vi "imu.vi"(4 "error in":errorcluster) -> (0 "error out":errorcluster, 1 "IMU configuration":string, 2 "Raw data":string, 3 "IMU Packet":T1 {"local_angular_velocity"."z" format="%#.4g"; "local_angular_velocity"."y" format="%#.4g"; "local_angular_velocity"."x" format="%#.4g"; "angular_acceleration"."z" format="%#.3g"; "angular_acceleration"."y" format="%#.3g"; "angular_acceleration"."x" format="%#.3g"; "orientation"."w" format="%#.4g"; "orientation"."z" format="%#.4g"; "orientation"."y" format="%#.4g"; "orientation"."x" format="%#.4g"; "position"."z" format="%#_5g"; "position"."y" format="%#_5g"; "position"."x" format="%#_5g"; "local_velocity"."z" format="%#.4g"; "local_velocity"."y" format="%#.4g"; "local_velocity"."x" format="%#.4g"; "local_acceleration"."z" format="%#.4g"; "local_acceleration"."y" format="%#.4g"; "local_acceleration"."x" format="%#.4g"; "velocity"."z" format="%#.3g"; "velocity"."y" format="%#.3g"; "velocity"."x" format="%#.3g"; "angular_velocity"."z" format="%#.4g"; "angular_velocity"."y" format="%#.4g"; "angular_velocity"."x" format="%#.4g"; "acceleration"."z" format="%#.4g"; "acceleration"."y" format="%#.4g"; "acceleration"."x" format="%#.4g"})   [LabVIEW 2019]
doc: "Reads and process the data stream for the IMU sensor. Outputs the IMU data in a cluster."
uses:
  tools/simx_common.vi
  controls/IMU_packet.ctl
  controls/Header.ctl
panel:
  out "Header":T2 {"game_time" format="%#_10g"}
  in  "IMU configuration":string="{\n    \"type\": \"IMU\",\n    \"listen_port\": 8500,\n    \"location\": {\n      \"x\": 50.0,\n      \"y\": 50.0,\n      \"z\": 50.0\n    },\n    \"rotation\": {\n      \"pitch\":0.0,\n      \"yaw\":0.0,\n      \"roll\":0.0\n    }\n  }"
  in  "null connection":refnum<k5>
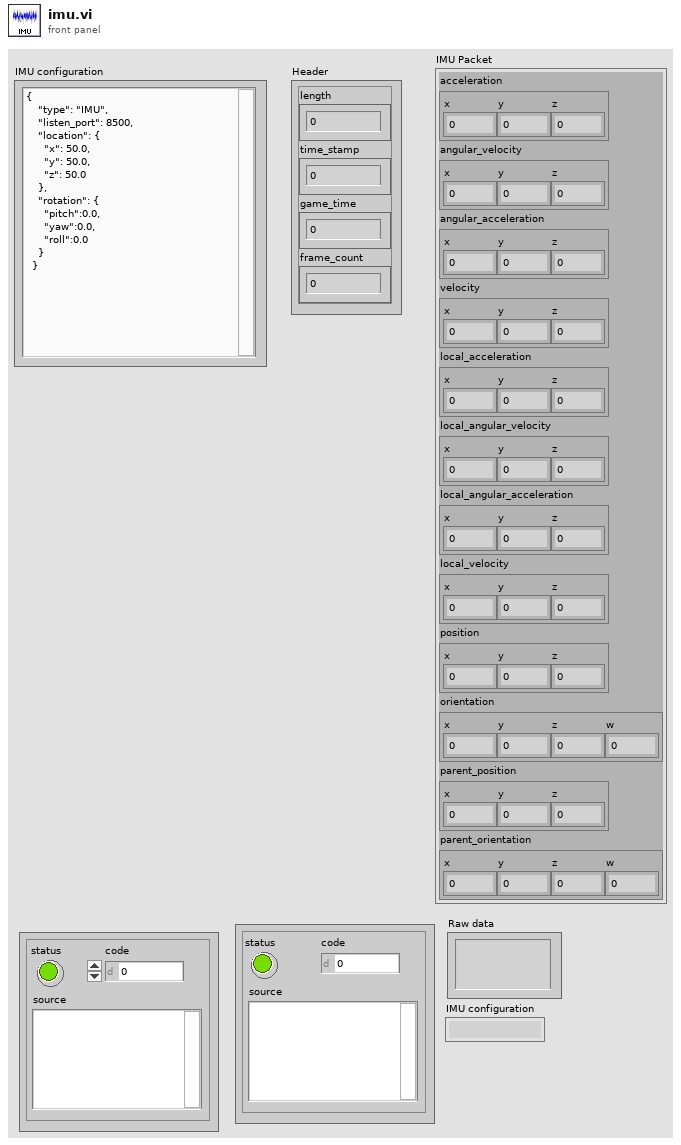
[diagram p1: front panel]
types:
  T1 = typedef "IMU_packet.ctl" = cluster{"acceleration":cluster{"x":sgl, "y":sgl, "z":sgl}, "angular_velocity":cluster{"x":sgl, "y":sgl, "z":sgl}, "angular_acceleration":cluster{"x":sgl, "y":sgl, "z":sgl}, "velocity ":cluster{"x":sgl, "y":sgl, "z":sgl}, "local_acceleration":cluster{"x":sgl, "y":sgl, "z":sgl}, "local_angular_velocity":cluster{"x":sgl, "y":sgl, "z":sgl}, "local_angular_acceleration":cluster{"x":sgl, "y":sgl, "z":sgl}, "local_velocity":cluster{"x":sgl, "y":sgl, "z":sgl}, "position":cluster{"x":sgl, "y":sgl, "z":sgl}, "orientation":cluster{"x":sgl, "y":sgl, "z":sgl, "w":sgl}, "parent_position":cluster{"x":sgl, "y":sgl, "z":sgl}, "parent_orientation":cluster{"x":sgl, "y":sgl, "z":sgl, "w":sgl}}
  T2 = typedef "Header.ctl" = cluster{"length":u32, "time_stamp":u32, "game_time":sgl, "frame_count":u32}
  T3 = typedef "simx_connection.ctl" = cluster{"Config":T4, "Connections":T7, "Map":cluster{"lanes":cluster{"x":dbl[], "y":dbl[], "z":dbl[]}, "StartPosition":cluster{"start_points":T8, "StartRotation":dbl[], "StartLocation":dbl[]}, "Draw Map Size":T9, "DrawArea":cluster{"min_Y":dbl, "min_X":dbl, "Scale X":dbl, "Scale Y":dbl}, "Map":picture, "Map Geojson":string}}
  T4 = typedef "config.ctl" = cluster{"Trajectory":T5, "Weather":T6}
  T5 = typedef "trajectory.ctl" = cluster{"Number of frames":i32, "Frame number":i32, "Trajectory":string}
  T6 = typedef "weather.ctl" = cluster{"id":string}
  T7 = typedef "connections.ctl" = cluster{"Simulator Connection":refnum<k5>, "server_ip":string, "Port":i32, "Sensor connections":refnum<k5>[]}
  T8 = typedef "start_points.ctl" = cluster{"locations":dbl[][], "rotations":dbl[][], "type":string[]}
  T9 = typedef "LVBoundsTypeDef.ctl" = cluster{"Width":u32, "Height":u32}
  T10 = enum16{"big-endian, network order", "native, host order", "little-endian"}
  T11 = typedef "sensor_sample.ctl" = cluster{"Header":T2, "data out":string}
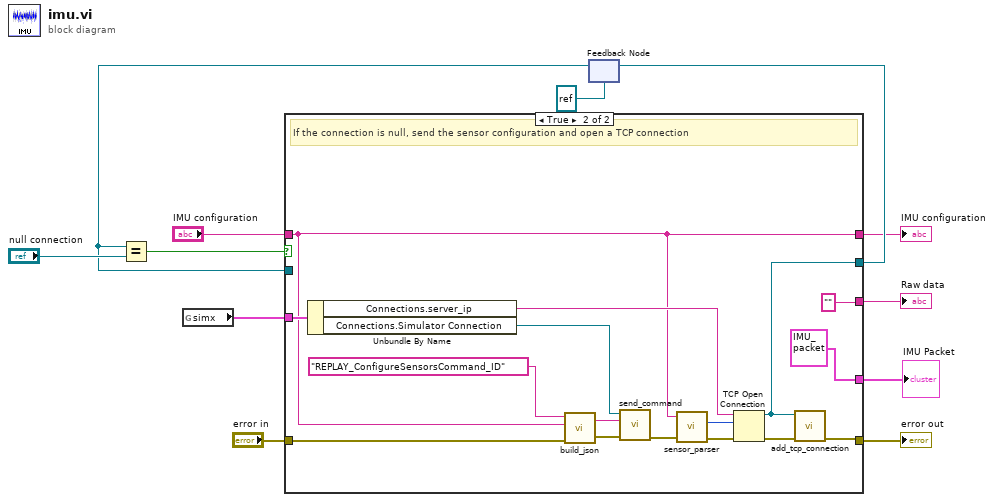
[diagram p0: block diagram]
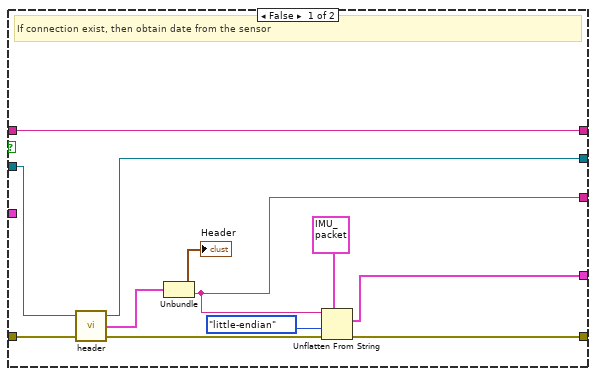
[diagram p2: hidden frame]
diagram:
  n1 = global read "simx_common.vi" "simx"() -> (w3:T3)
  n2 = feedback #1(refnum<k5> refnum ("connection ID")) -> (w7:refnum<k5>)
  n3 = Equal?(x=w7, y="null connection") -> (x = y?=w8:bool)
  n4 = case shown="True" w8 {
    tunnel: [w20 w27] -> w12
    tunnel: "IMU configuration" -> [w17 w28]
    tunnel: [w21 w26] -> w9
    tunnel: w7 -> [w19 _]
    tunnel: "error in" -> [w22 w35]
    tunnel: [w18 "" ("data out")] -> w5
    tunnel: [w17 w28] -> w4
    tunnel: w3 -> [_ w33]
    tunnel: [w14 T1 {"acceleration"={"x"=0.0, "y"=0.0, "z"=0.0}, "angular_velocity"={"x"=0.0, "y"=0.0, "z"=0.0}, "angular_acceleration"={"x"=0.0, "y"=0.0, "z"=0.0}, "velocity "={"x"=0.0, "y"=0.0, "z"=0.0}, "local_acceleration"={"x"=0.0, "y"=0.0, "z"=0.0}, "local_angular_velocity"={"x"=0.0, "y"=0.0, "z"=0.0}, "local_angular_acceleration"={"x"=0.0, "y"=0.0, "z"=0.0}, "local_velocity"={"x"=0.0, "y"=0.0, "z"=0.0}, "position"={"x"=0.0, "y"=0.0, "z"=0.0}, "orientation"={"x"=0.0, "y"=0.0, "z"=0.0, "w"=0.0}, "parent_position"={"x"=0.0, "y"=0.0, "z"=0.0}, "parent_orientation"={"x"=0.0, "y"=0.0, "z"=0.0, "w"=0.0}} ("IMU Packet")] -> w1
    frame False {
      # "If connection exist, then obtain date from the sensor"
      n5 = call "header.vi"("error in"=w22, "TCP Network Connection in"=w19) -> ("error out"=w23:errorcluster, "Sensor sample"=w24:T11, "TCP Network Connection out"=w21:refnum<k5>)  [unwired: 1 in]
      n6 = Unbundle(w24) -> ("Header"=→"Header":T2, "data out"=w18:string)
      n7 = Unflatten From String(type=T1 {"acceleration"={"x"=0.0, "y"=0.0, "z"=0.0}, "angular_velocity"={"x"=0.0, "y"=0.0, "z"=0.0}, "angular_acceleration"={"x"=0.0, "y"=0.0, "z"=0.0}, "velocity "={"x"=0.0, "y"=0.0, "z"=0.0}, "local_acceleration"={"x"=0.0, "y"=0.0, "z"=0.0}, "local_angular_velocity"={"x"=0.0, "y"=0.0, "z"=0.0}, "local_angular_acceleration"={"x"=0.0, "y"=0.0, "z"=0.0}, "local_velocity"={"x"=0.0, "y"=0.0, "z"=0.0}, "position"={"x"=0.0, "y"=0.0, "z"=0.0}, "orientation"={"x"=0.0, "y"=0.0, "z"=0.0, "w"=0.0}, "parent_position"={"x"=0.0, "y"=0.0, "z"=0.0}, "parent_orientation"={"x"=0.0, "y"=0.0, "z"=0.0, "w"=0.0}} ("IMU Packet"), binary string=w18, byte order (0:big-endian, network order)=T10."little-endian", error in (no error)=w23) -> (value=w14:T1, error out=w20:errorcluster)  [unwired: 1 in, 1 out]
    }
    frame True {
      # "If the connection is null, send the sensor configuration and open a TCP connection"
      n8 = Unbundle By Name(w33) -> ("Connections.server_ip"=w31:string, "Connections.Simulator Connection"=w32:refnum<k5>)
      n9 = call "build_json.vi"("error in"=w35, "Message"=w28, "Command_ID"="REPLAY_ConfigureSensorsCommand_ID") -> ("error out"=w38:errorcluster, "JSON Out"=w39:string)  [unwired: 1 in]
      n10 = call "send_command.vi"("error in"=w38, "JSON Command"=w39, "TCP Network Connection in"=w32) -> ("error out"=w37:errorcluster)  [unwired: 1 in, 3 out]
      n11 = call "sensor_parser.vi"("Sensor configuration"=w28, "error in"=w37) -> ("Port out"=w29:u16, "error out"=w30:errorcluster)  [unwired: 1 in, 2 out]
      n12 = TCP Open Connection(address=w31, remote port or service name=w29, error in (no error)=w30) -> (connection ID=w26:refnum<k5>, error out=w36:errorcluster)  [unwired: 2 in]
      n13 = call "add_tcp_connection.vi"("error in"=w36, "Sensor connection"=w26) -> ("error out"=w27:errorcluster)  [unwired: 5 in]
    }
  }
  "error out" <- w12
  "Raw data" <- w5
  "IMU configuration" <- w4
  "IMU Packet" <- w1
  n14 = feedback-in #1(w9) -> ()
